vi "Value (DBL).vi"(10 "error in (no error)":errorcluster, 11 "Config Element in":refnum<class "Config Element.lvclass">) -> (2 "error out":errorcluster, 3 "DBL Value":dbl)   [LabVIEW 2020, in "CDM-Config.lvlib" / "Config Element.lvclass"]
uses:
  Config Element.lvclass
  Config Element.lvclass/Config Element.ctl
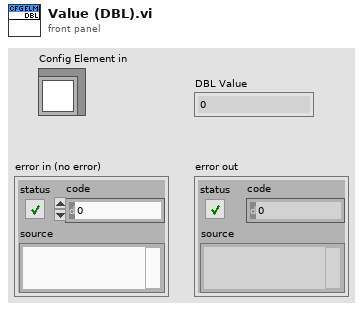
[diagram p1: front panel]
types:
  T1 = typedef "CDM-Config.lvlib/Config Element.lvclass/Ref Data.ctl" = cluster{"Node Info":T2, "Owner":refnum<class>, "Changed":bool, "Name":string, "Meta Data":T3[], "Array":bool, "Value Type":T4, "Value":variant}
  T2 = typedef "CDM-Config.lvlib/Node Info.ctl" = cluster{"Index":i32, "Parent":i32, "Children":i32[]}
  T3 = typedef "CDM-Config.lvlib/Meta Data.ctl" = cluster{"Name":string, "Value":string}
  T4 = typedef "CDM-Config.lvlib/Value Type.ctl" = enum16{"String", "Number", "Bool", "Object", "Array"}
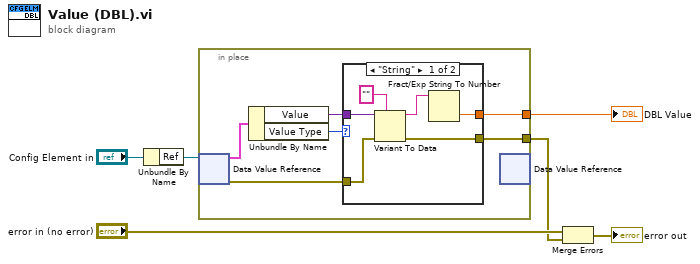
[diagram p0: block diagram]
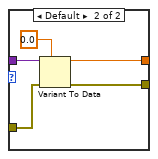
[diagram p2: hidden frame]
diagram:
  n1 = Unbundle By Name("Config Element in") -> ("Ref"=w3:refnum<data-value>)
  n2 = in-place {
    in-place-border: [w8] -> w2
    in-place-border: [w7] -> w1
    n3 = in-place-dvr #1(w3) -> (w12:T1, w11:errorcluster)
    n4 = Unbundle By Name(w12) -> ("Value"=w9:variant, "Value Type"=w10:T4)
    n5 = case shown="\"String\"" w10 {
      tunnel: w11 -> [w17 w20]
      tunnel: w9 -> [w18 w23]
      tunnel: [w13 w21] -> w8
      tunnel: [w16 w19] -> w7
      frame "String" {
        n6 = Variant To Data(error in=w17, type="", Variant=w18) -> (data=w14:string, error out=w16:errorcluster)
        n7 = Fract/Exp String To Number(string=w14) -> (number=w13:dbl)  [unwired: 3 in, 1 out]
      }
      frame Default {
        n8 = Variant To Data(error in=w20, type=0.0, Variant=w23) -> (data=w21:dbl, error out=w19:errorcluster)
      }
    }
    n9 = in-place-dvr #1() -> ()  [unwired: 1 in, 2 out]
  }
  "DBL Value" <- w2
  n10 = Merge Errors("error in (no error)", w1) -> (→"error out":errorcluster)
